vi "Remove RTV [by name].vi"(0 "RTV name":string, 11 "error in (no error)":errorcluster) -> (15 "error out":errorcluster)   [LabVIEW 2016, in "RT Variables.lvclass"]
uses:
  RT Variables.lvclass
  protected/Singleton Action.ctl
  RT Variables.lvclass/RT Variables.ctl
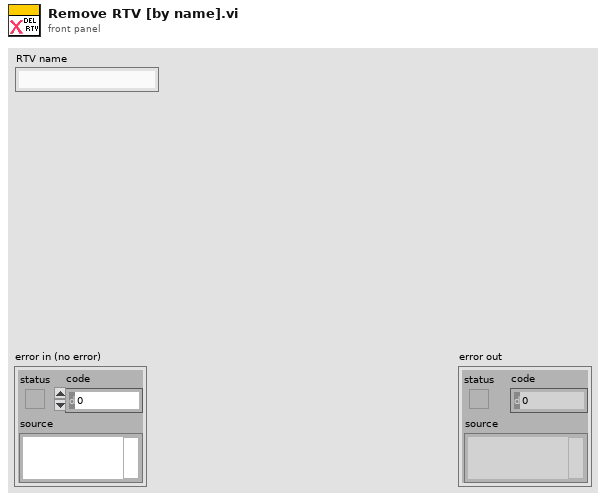
[diagram p1: front panel]
types:
  T1 = typedef "RT Variables.lvclass/Singleton Action.ctl" = enum16{"Get", "Set"}
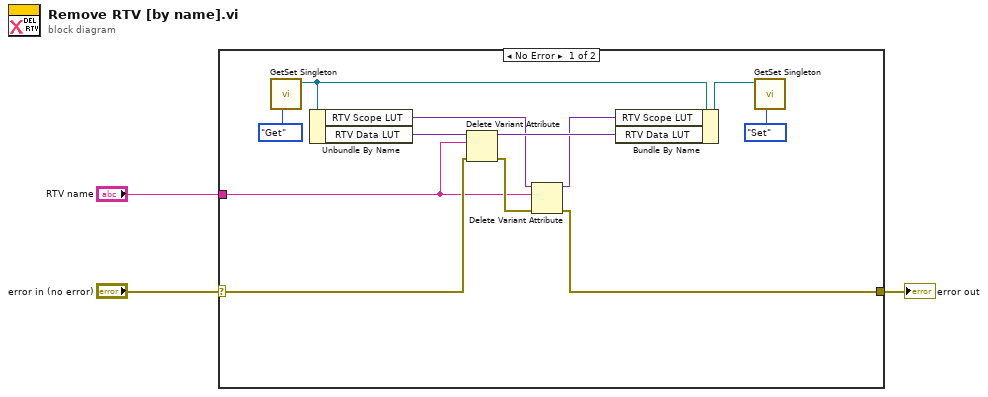
[diagram p0: block diagram]
diagram:
  n1 = case shown="No Error" "error in (no error)" {
    selector: "error in (no error)" -> [w9 w16]
    tunnel: [w5 w16] -> w2
    tunnel: "RTV name" -> [w4 _]
    frame No Error {
      n2 = call "GetSet Singleton.vi"("Action"=Singleton_Action."Get") -> ("RT Variables out"=w13:refnum<class "RT Variables.lvclass">)  [unwired: 9 in, 1 out]
      n3 = Unbundle By Name(w13) -> ("RTV Scope LUT"=w8:variant, "RTV Data LUT"=w11:variant)
      n4 = Delete Variant Attribute(4:w9, 6:w4, 7:w11) -> (0:w6:errorcluster, 3:w10:variant)  [unwired: 1 out]
      n5 = Delete Variant Attribute(4:w6, 6:w4, 7:w8) -> (0:w5:errorcluster, 3:w7:variant)  [unwired: 1 out]
      n6 = Bundle By Name(cluster=w13, "RTV Scope LUT"=w7, "RTV Data LUT"=w10) -> (w12:refnum<class "RT Variables.lvclass">)
      n7 = call "GetSet Singleton.vi"("Action"=Singleton_Action."Set", "RT Variables in"=w12) -> ()  [unwired: 8 in, 2 out]
    }
    frame Error {
    }
  }
  "error out" <- w2
